vi "MagnetoCaloricSweep.vi"() -> ()   [LabVIEW 2019]
uses:
  Instrument_Setup.vi
  Global/Global Variables/Heat_global_variables.vi
  Global/Global Variables/Data_Display_global.vi
  Global/Global Variables/global.vi
  Equipment/Lake Shore 372/Lake Shore 372.lvlib
panel:
  out "Time":u32[](array[numeric])
  out "Indices":i32[](array[numeric])
  out "Bath Temperature":dbl[](array[numeric])
  out "Sample temperatur":dbl[](array[numeric])
  out "XY Graph":cluster{dbl[], dbl[]}[](graph)
  out "Wait":bool
  out "R2":dbl
  out "T2":dbl
  out "T1":dbl
  out "R1":dbl
  in  "Measure for (s)":dbl=5.0
  out "Was LS370_readout-Monitor activatet?":bool
  out "Was LS372_readout-Monitor activatet?":bool
  out "Was K2182A-Monitor activatet?":bool
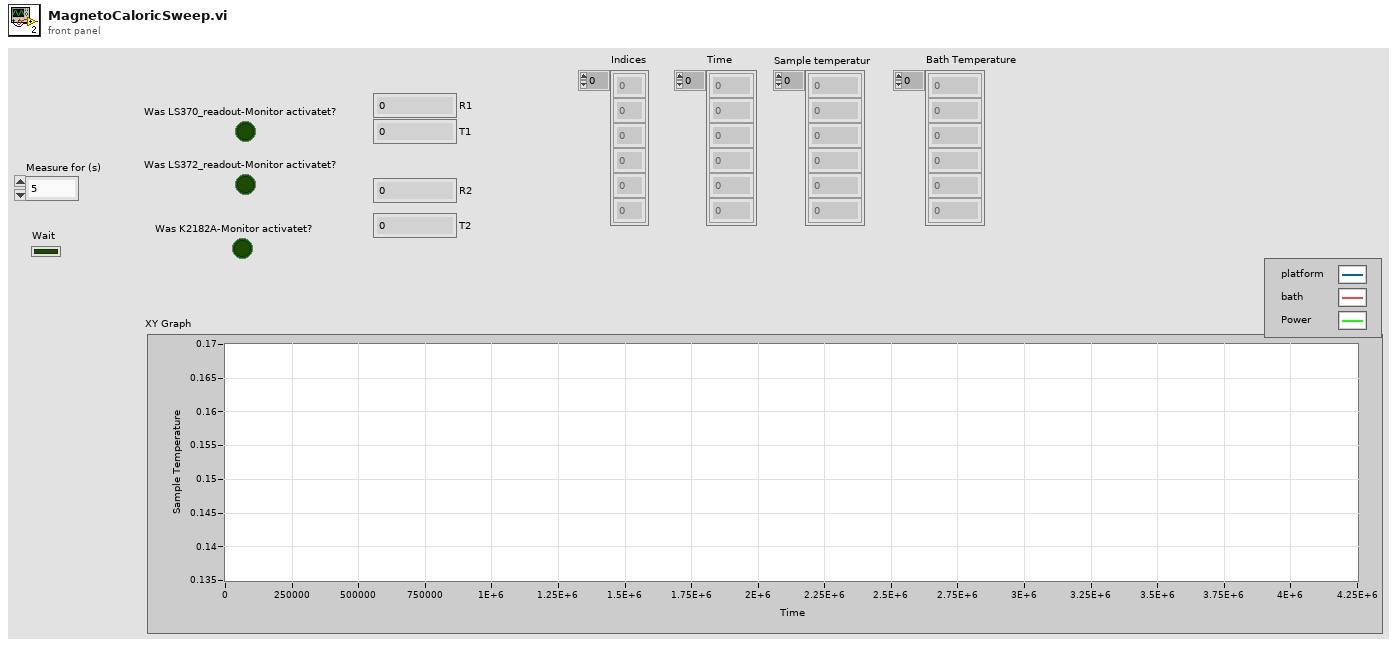
[diagram p1: front panel]
types:
  T1 = cluster{"Lakeshore 370 ":refnum<visa-resource-name>, "Lakeshore 372":refnum<visa-resource-name>, "Platform Channel":i32, "Bath Channel ":i32, "Platform Temperature Control":u16, "Bath Temperature Control":u16}
  T2 = typedef "AMI_cluster.ctl" = cluster{"Y Axis Status":enum16{"", "RAMPING", "HOLDING", "PAUSED", "MANUAL UP", "MANUAL DOWN", "ZEROING CURRENT", "QUENCH DETECTED", "HEATING SWITCH", "AT ZER0", "COOLING SWITCH"}, "Z Axis Status":enum16{"", "RAMPING", "HOLDING", "PAUSED", "MANUAL UP", "MANUAL DOWN", "ZEROING CURRENT", "QUENCH DETECTED", "HEATING SWITCH", "AT ZER0", "COOLING SWITCH"}, "Y-Axis (T)":dbl, "Y-Axis Setpoint (T)":dbl, "Y-Axis Rate (T/min)":dbl, "Z-Axis (T)":dbl, "Z-Axis Setpoint (T)":dbl, "Z-Axis Rate (T/min)":dbl, "B AMI rate (T)":dbl, "AMI Monitor":bool, "AMI Set field rates":bool, "AMI Set field":bool, "Switch Heater Y":bool, "Switch Heater Z":bool, "Switch Heater":bool, "B AMI (T)":dbl, "B AMI Setpoint (T)":dbl, "Phi AMI (Deg) ":dbl, "Phi AMI Setpoint (Deg) ":dbl}
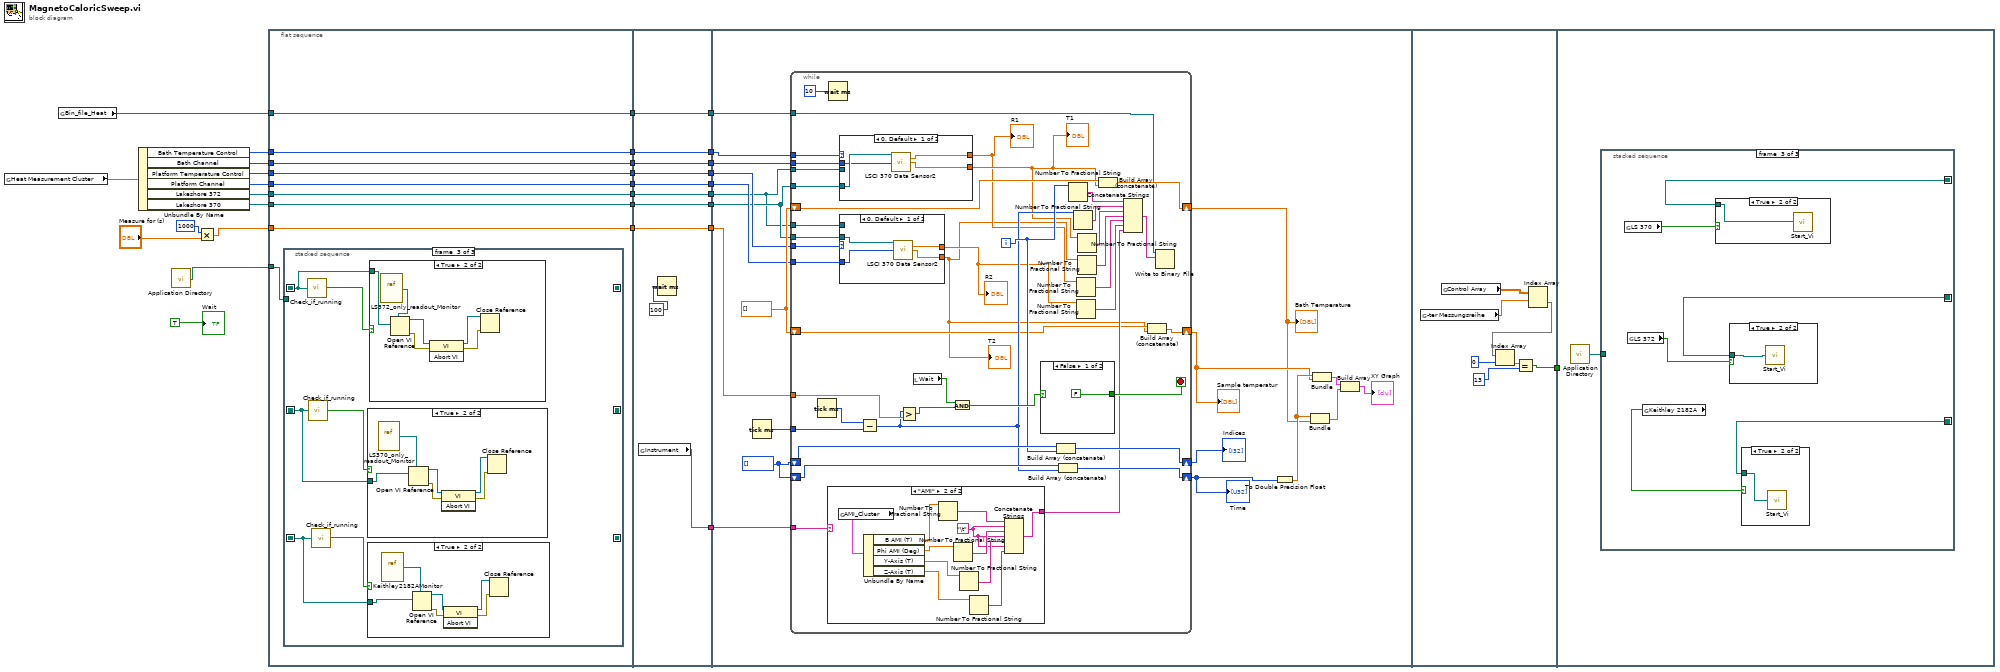
[diagram p0: block diagram]
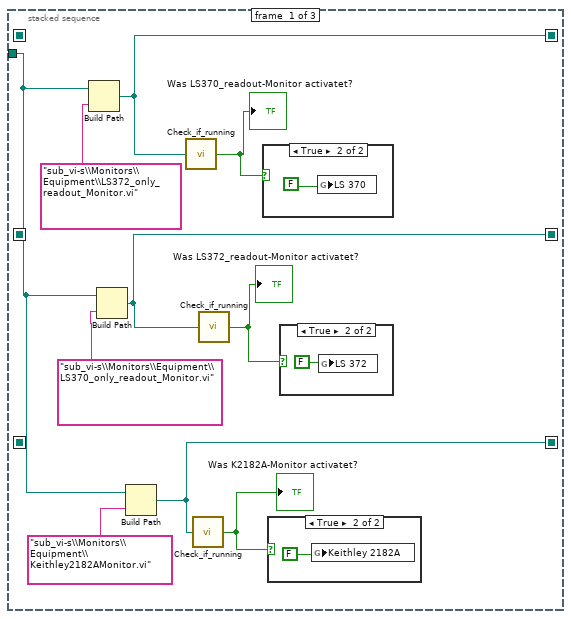
[diagram p2: hidden frame]
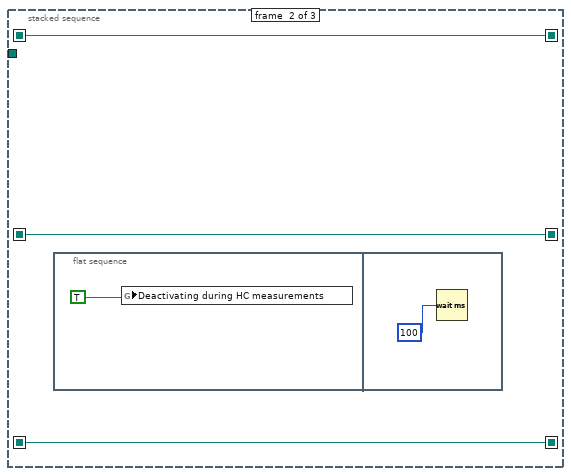
[diagram p6: hidden frame]
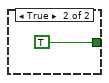
[diagram p10: hidden frame]
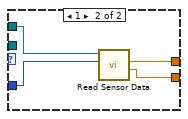
[diagram p11: hidden frame]
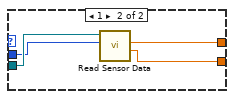
[diagram p12: hidden frame]
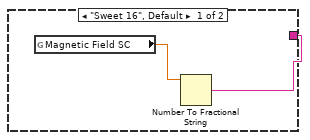
[diagram p13: hidden frame]
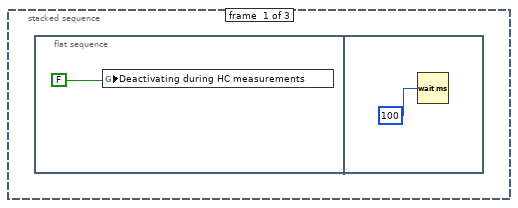
[diagram p14: hidden frame]
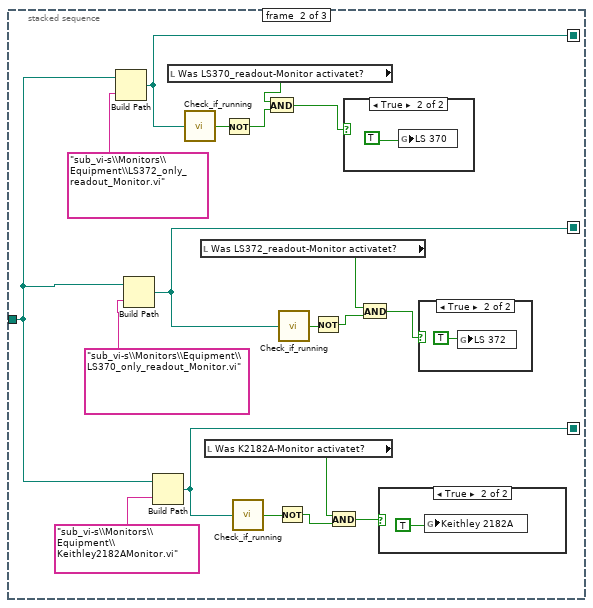
[diagram p15: hidden frame]
diagram:
  n1 = global read "Instrument_Setup.vi" "Heat Measurement Cluster"() -> (w31:T1)
  n2 = global read "Heat_global_variables.vi" "Bin_file_Heat"() -> (w23:refnum<file>)
  n3 = Unbundle By Name(w31) -> ("Bath Temperature Control"=w30:u16, "Bath Channel"=w29:i32, "Platform Temperature Control"=w28:u16, "Platform Channel"=w27:i32, "Lakeshore 372"=w26:refnum<visa-resource-name>, "Lakeshore 370"=w25:refnum<visa-resource-name>)
  n4 = call <vilib>:"Application Directory.vi"() -> ("Application Directory"=w24:path)
  n5 = Multiply(x=1000, y="Measure for (s)") -> (x*y=w20:dbl)
  n6 = flat-sequence {
    tunnel: w30 -> [w38]
    tunnel: w29 -> [w37]
    tunnel: w28 -> [w36]
    tunnel: w27 -> [w35]
    tunnel: w26 -> [w34]
    tunnel: w25 -> [w33]
    tunnel: w24 -> [w40]
    tunnel: w23 -> [w39]
    tunnel: w20 -> [w32]
    tunnel: [w39] -> w19
    tunnel: [w38] -> w18
    tunnel: [w37] -> w17
    tunnel: [w36] -> w16
    tunnel: [w35] -> w15
    tunnel: [w34] -> w14
    tunnel: [w33] -> w13
    tunnel: [w32] -> w12
    tunnel: w19 -> [w84]
    tunnel: w18 -> [w90]
    tunnel: w17 -> [w89]
    tunnel: w16 -> [w88]
    tunnel: w15 -> [w87]
    tunnel: w14 -> [w86]
    tunnel: w13 -> [w92]
    tunnel: w12 -> [w91]
    tunnel: [w92] -> w11
    tunnel: [w91] -> w10
    tunnel: [w90] -> w9
    tunnel: [w89] -> w8
    tunnel: [w88] -> w7
    tunnel: [w87] -> w6
    tunnel: [w86] -> w5
    tunnel: [w84] -> w4
    tunnel: [w83] -> w3
    tunnel: w11 -> [w102]
    tunnel: w10 -> [w108]
    tunnel: w9 -> [w107]
    tunnel: w8 -> [w106]
    tunnel: w7 -> [w104]
    tunnel: w6 -> [w103]
    tunnel: w5 -> [w101]
    tunnel: w4 -> [w105]
    tunnel: w3 -> [w112]
    tunnel: [w184] -> w1
    tunnel: w1 -> [_]
    frame #0 {
      n7 = stacked-sequence {
        seq-local: [w43 _ _] -> [_ w56 _]
        seq-local: [w42 _ _] -> [_ w55 _]
        seq-local: [w41 _ _] -> [_ w54 _]
        seq-local: [_ w56 _] -> [_ _ w61]
        seq-local: [_ w55 _] -> [_ _ w60]
        seq-local: [_ w54 _] -> [_ _ w59]
        tunnel: w40 -> [w48 _ _]
        frame #0 {
          n8 = Build Path(base path=w48, name or relative path="sub_vi-s\\Monitors\\Equipment\\LS372_only_readout_Monitor.vi") -> (appended path=w43:path)
          n9 = Build Path(base path=w48, name or relative path="sub_vi-s\\Monitors\\Equipment\\LS370_only_readout_Monitor.vi") -> (appended path=w42:path)
          n10 = Build Path(base path=w48, name or relative path="sub_vi-s\\Monitors\\Equipment\\Keithley2182AMonitor.vi") -> (appended path=w41:path)
          n11 = call "Check_if_running.vi"("VI-Pfad"=w43) -> ("Running"=w46:bool)
          "Was LS370_readout-Monitor activatet?" <- w46
          n12 = call "Check_if_running.vi"("VI-Pfad"=w41) -> ("Running"=w44:bool)
          "Was K2182A-Monitor activatet?" <- w44
          n13 = call "Check_if_running.vi"("VI-Pfad"=w42) -> ("Running"=w45:bool)
          "Was LS372_readout-Monitor activatet?" <- w45
          n14 = case shown="True" w46 {
            frame False {
            }
            frame True {
              n15 = global write "Instrument_Setup.vi" "LS 370"(FALSE) -> ()
            }
          }
          n16 = case shown="True" w44 {
            frame False {
            }
            frame True {
              n17 = global write "Instrument_Setup.vi" "Keithley 2182A"(FALSE) -> ()
            }
          }
          n18 = case shown="True" w45 {
            frame False {
            }
            frame True {
              n19 = global write "Instrument_Setup.vi" "LS 372"(FALSE) -> ()
            }
          }
        }
        frame #1 {
          n20 = flat-sequence {
            frame #0 {
              n21 = global write "Data_Display_global.vi" "Deactivating during HC measurements"(TRUE) -> ()
            }
            frame #1 {
              n22 = Wait (ms)(milliseconds to wait=100) -> ()  [unwired: 1 out]
            }
          }
        }
        frame #2 {
          n23 = call "Check_if_running.vi"("VI-Pfad"=w61) -> ("Running"=w64:bool)
          n24 = call "Check_if_running.vi"("VI-Pfad"=w60) -> ("Running"=w63:bool)
          n25 = call "Check_if_running.vi"("VI-Pfad"=w59) -> ("Running"=w62:bool)
          n26 = case shown="True" w63 {
            tunnel: w60 -> [_ w76]
            frame False {
            }
            frame True {
              n27 = vi-ref "LS370_only_readout_Monitor.vi"() -> (w75:refnum<vi>)
              n28 = Open VI Reference(type specifier VI Refnum (for type only)=w75, vi path=w76) -> (vi reference=w74:refnum<vi>, error out=w73:errorcluster)  [unwired: 4 in]
              n29 = invoke class="VI" method="Abort VI"(reference=w74, error in=w73) -> (reference out=w72:refnum<vi>, error out=w71:errorcluster)  [unwired: 1 in, 1 out]
              n30 = Close Reference(reference=w72, error in (no error)=w71) -> ()  [unwired: 1 out]
            }
          }
          n31 = case shown="True" w62 {
            tunnel: w59 -> [_ w70]
            frame False {
            }
            frame True {
              n32 = vi-ref "Keithley2182AMonitor.vi"() -> (w69:refnum<vi>)
              n33 = Open VI Reference(type specifier VI Refnum (for type only)=w69, vi path=w70) -> (vi reference=w68:refnum<vi>, error out=w67:errorcluster)  [unwired: 4 in]
              n34 = invoke class="VI" method="Abort VI"(reference=w68, error in=w67) -> (reference out=w66:refnum<vi>, error out=w65:errorcluster)  [unwired: 1 in, 1 out]
              n35 = Close Reference(reference=w66, error in (no error)=w65) -> ()  [unwired: 1 out]
            }
          }
          n36 = case shown="True" w64 {
            tunnel: w61 -> [_ w81]
            frame False {
            }
            frame True {
              n37 = vi-ref "LS372_only_readout_Monitor.vi"() -> (w82:refnum<vi>)
              n38 = Open VI Reference(type specifier VI Refnum (for type only)=w82, vi path=w81) -> (vi reference=w80:refnum<vi>, error out=w79:errorcluster)  [unwired: 4 in]
              n39 = invoke class="VI" method="Abort VI"(reference=w80, error in=w79) -> (reference out=w78:refnum<vi>, error out=w77:errorcluster)  [unwired: 1 in, 1 out]
              n40 = Close Reference(reference=w78, error in (no error)=w77) -> ()  [unwired: 1 out]
            }
          }
        }
      }
    }
    frame #1 {
      n41 = global read "Instrument_Setup.vi" "Instrument"() -> (w83:string)
      n42 = Wait (ms)(milliseconds to wait=100) -> ()  [unwired: 1 out]
    }
    frame #2 {
      w109 = dbl[] []
      w110 = i32[] []
      n43 = Tick Count (ms)() -> (millisecond timer value=w111:u32)
      n44 = while {
        tunnel: w112 -> [w152]
        tunnel: w111 -> [w150]
        shift-right: [w142] -> w100
        shift-left: w110 -> [w143]
        shift-right: [w140] -> w99
        shift-left: w110 -> [w141]
        shift-right: [w138] -> w96
        shift-left: w109 -> [w139]
        shift-right: [w114] -> w97
        shift-left: w109 -> [w115]
        tunnel: w108 -> [w149]
        tunnel: w107 -> [w147]
        tunnel: w101 -> [w146]
        tunnel: w102 -> [w145]
        tunnel: w106 -> [w144]
        tunnel: w105 -> [w129]
        tunnel: w104 -> [w137]
        tunnel: w103 -> [w136]
        tunnel: w102 -> [w135]
        tunnel: w101 -> [w134]
        i -> [w128]
        stop <- w130 stop-if-true
        n45 = Tick Count (ms)() -> (millisecond timer value=w151:u32)
        n46 = case shown="\"AMI\"" w152 {
          tunnel: [w171 w181] -> w117
          frame "Sweet 16", Default {
            n47 = global read "Data_Display_global.vi" "Magnetic Field SC"() -> (w172:dbl)
            n48 = Number To Fractional String(number=w172) -> (F-format string=w171:string)  [unwired: 3 in]
          }
          frame "AMI" {
            w178 = "\t"
            n49 = global read "Data_Display_global.vi" "AMI_Cluster"() -> (w177:T2)
            n50 = Unbundle By Name(w177) -> ("B AMI (T)"=w176:dbl, "Phi AMI (Deg)"=w175:dbl, "Y-Axis (T)"=w174:dbl, "Z-Axis (T)"=w173:dbl)
            n51 = Number To Fractional String(number=w176) -> (F-format string=w183:string)  [unwired: 3 in]
            n52 = Number To Fractional String(number=w175) -> (F-format string=w182:string)  [unwired: 3 in]
            n53 = Number To Fractional String(number=w174) -> (F-format string=w180:string)  [unwired: 3 in]
            n54 = Number To Fractional String(number=w173) -> (F-format string=w179:string)  [unwired: 3 in]
            n55 = Concatenate Strings(w183, w178, w182, w178, w180, w178, w179) -> (w181:string)
          }
        }
        n56 = Wait (ms)(milliseconds to wait=10) -> ()  [unwired: 1 out]
        n57 = case shown="0, Default" w147 {
          tunnel: w146 -> [_ w170]
          tunnel: w145 -> [w166 _]
          tunnel: w144 -> [w165 w169]
          tunnel: [w164 w168] -> w121
          tunnel: [w163 w167] -> w124
          frame 0, Default {
            n58 = call "LSCI 370 Data Sensor2.vi"("VISA session"=w166, "Channel (1)"=w165) -> ("Resistance Reading"=w164:dbl, "Kelvin Reading"=w163:dbl)  [unwired: 9 in, 3 out]
          }
          frame 1 {
            n59 = call "Read Sensor Data.vi"("Channel (1:1)"=w169, "VISA resource name"=w170) -> ("Kelvin Reading"=w167:dbl, "Resistance Reading"=w168:dbl)  [unwired: 4 in, 4 out]
          }
        }
        "R1" <- w121
        "T1" <- w124
        n60 = case shown="0, Default" w137 {
          tunnel: w136 -> [w155 w161]
          tunnel: w135 -> [w156 _]
          tunnel: w134 -> [_ w162]
          tunnel: [w158 w160] -> w119
          tunnel: [w157 w159] -> w113
          frame 0, Default {
            n61 = call "LSCI 370 Data Sensor2.vi"("VISA session"=w156, "Channel (1)"=w155) -> ("Resistance Reading"=w158:dbl, "Kelvin Reading"=w157:dbl)  [unwired: 9 in, 3 out]
          }
          frame 1 {
            n62 = call "Read Sensor Data.vi"("Channel (1:1)"=w161, "VISA resource name"=w162) -> ("Kelvin Reading"=w159:dbl, "Resistance Reading"=w160:dbl)  [unwired: 4 in, 4 out]
          }
        }
        "T2" <- w113
        "R2" <- w119
        n63 = Subtract(x=w151, y=w150) -> (x-y=w126:u32)
        n64 = Greater?(x=w126, y=w149) -> (0:w133:bool)
        n65 = local read "Wait"() -> (w132:bool)
        n66 = And(x=w132, y=w133) -> (x .and. y?=w131:bool)
        n67 = case shown="False" w131 {
          tunnel: [FALSE TRUE] -> w130
          frame False {
          }
          frame True {
          }
        }
        n68 = Build Array (concatenate)(w143, w128) -> (w142:i32[])
        n69 = Build Array (concatenate)(w141, w126) -> (w140:u32[])
        n70 = Number To Fractional String(number=w128) -> (F-format string=w127:string)  [unwired: 3 in]
        n71 = Number To Fractional String(number=w126) -> (F-format string=w125:string)  [unwired: 3 in]
        n72 = Number To Fractional String(number=w121) -> (F-format string=w120:string)  [unwired: 3 in]
        n73 = Number To Fractional String(number=w119) -> (F-format string=w118:string)  [unwired: 3 in]
        n74 = Number To Fractional String(number=w113) -> (F-format string=w122:string)  [unwired: 3 in]
        n75 = Number To Fractional String(number=w124) -> (F-format string=w123:string)  [unwired: 3 in]
        n76 = Build Array (concatenate)(w139, w124) -> (w138:dbl[])
        n77 = Concatenate Strings(w127, w125, w123, w122, w120, w118, w117) -> (w116:string)
        n78 = Build Array (concatenate)(w115, w113) -> (w114:dbl[])
        n79 = Write to Binary File(file (use dialog)=w129, data=w116) -> ()  [unwired: 4 in, 3 out]
      }
      "Sample temperatur" <- w97
      "Bath Temperature" <- w96
      "Indices" <- w100
      "Time" <- w99
      n80 = To Double Precision Float(number=w99) -> (double precision float=w98:dbl[])
      n81 = Bundle(w98, w96) -> (w94:cluster{dbl[], dbl[]})  [unwired: 1 in]
      n82 = Bundle(w98, w97) -> (w95:cluster{dbl[], dbl[]})  [unwired: 1 in]
      n83 = Build Array(w95, w94) -> (→"XY Graph":cluster{dbl[], dbl[]}[])
    }
    frame #3 {
      n84 = global read "global.vi" "-ter Messungsreihe"() -> (w190:dbl)
      n85 = global read "global.vi" "Control Array"() -> (w188:dbl[][])
      n86 = Index Array(array=w188, index (row)=w190) -> (element=w189:dbl[])  [unwired: 1 in]
      n87 = Index Array(array=w189, index=0) -> (element=w186:dbl)
      n88 = Equal?(x=w186, y=13) -> (x = y?=w184:bool)
    }
    frame #4 {
      n89 = call <vilib>:"Application Directory.vi"() -> ("Application Directory"=w191:path)
      n90 = stacked-sequence {
        seq-local: [_ w204 _] -> [_ _ w218]
        seq-local: [_ w200 _] -> [_ _ w217]
        seq-local: [_ w195 _] -> [_ _ w216]
        tunnel: w191 -> [_ w209 _]
        frame #0 {
          n91 = flat-sequence {
            frame #0 {
              n92 = global write "Data_Display_global.vi" "Deactivating during HC measurements"(FALSE) -> ()
            }
            frame #1 {
              n93 = Wait (ms)(milliseconds to wait=100) -> ()  [unwired: 1 out]
            }
          }
        }
        frame #1 {
          n94 = Build Path(base path=w209, name or relative path="sub_vi-s\\Monitors\\Equipment\\LS372_only_readout_Monitor.vi") -> (appended path=w204:path)
          n95 = Build Path(base path=w209, name or relative path="sub_vi-s\\Monitors\\Equipment\\LS370_only_readout_Monitor.vi") -> (appended path=w200:path)
          n96 = Build Path(base path=w209, name or relative path="sub_vi-s\\Monitors\\Equipment\\Keithley2182AMonitor.vi") -> (appended path=w195:path)
          n97 = local read "Was LS370_readout-Monitor activatet?"() -> (w205:bool)
          n98 = call "Check_if_running.vi"("VI-Pfad"=w204) -> ("Running"=w208:bool)
          n99 = local read "Was LS372_readout-Monitor activatet?"() -> (w199:bool)
          n100 = local read "Was K2182A-Monitor activatet?"() -> (w194:bool)
          n101 = Not(x=w208) -> (.not. x?=w207:bool)
          n102 = call "Check_if_running.vi"("VI-Pfad"=w195) -> ("Running"=w197:bool)
          n103 = And(x=w205, y=w207) -> (x .and. y?=w206:bool)
          n104 = Not(x=w197) -> (.not. x?=w196:bool)
          n105 = call "Check_if_running.vi"("VI-Pfad"=w200) -> ("Running"=w203:bool)
          n106 = Not(x=w203) -> (.not. x?=w202:bool)
          n107 = And(x=w194, y=w196) -> (x .and. y?=w198:bool)
          n108 = case shown="True" w206 {
            frame False {
            }
            frame True {
              n109 = global write "Instrument_Setup.vi" "LS 370"(TRUE) -> ()
            }
          }
          n110 = And(x=w199, y=w202) -> (x .and. y?=w201:bool)
          n111 = case shown="True" w198 {
            frame False {
            }
            frame True {
              n112 = global write "Instrument_Setup.vi" "Keithley 2182A"(TRUE) -> ()
            }
          }
          n113 = case shown="True" w201 {
            frame False {
            }
            frame True {
              n114 = global write "Instrument_Setup.vi" "LS 372"(TRUE) -> ()
            }
          }
        }
        frame #2 {
          n115 = global read "Instrument_Setup.vi" "LS 370"() -> (w221:bool)
          n116 = global read "Instrument_Setup.vi" "LS 372"() -> (w220:bool)
          n117 = global read "Instrument_Setup.vi" "Keithley 2182A"() -> (w219:bool)
          n118 = case shown="True" w221 {
            tunnel: w218 -> [_ w224]
            frame False {
            }
            frame True {
              n119 = call "Start_Vi.vi"("VI-Pfad"=w224) -> ()  [unwired: 1 in]
            }
          }
          n120 = case shown="True" w220 {
            tunnel: w217 -> [_ w223]
            frame False {
            }
            frame True {
              n121 = call "Start_Vi.vi"("VI-Pfad"=w223) -> ()  [unwired: 1 in]
            }
          }
          n122 = case shown="True" w219 {
            tunnel: w216 -> [_ w222]
            frame False {
            }
            frame True {
              n123 = call "Start_Vi.vi"("VI-Pfad"=w222) -> ()  [unwired: 1 in]
            }
          }
        }
      }
    }
  }
  "Wait" <- TRUE
